vi "Read Config.vi"(8 "error in (no error)":errorcluster, 9 "Re-Init?":bool, 10 "ICM File In":path, 11 "Scaling in":refnum<class "Scaling.lvclass">) -> (0 "error out":errorcluster, 3 "Scaling out":refnum<class "Scaling.lvclass">)   [LabVIEW 2018, in "Scaling.lvclass"]
doc: "Scaling.lvclass:Read Config.vi\n\nThis is the template for the Read Config VI for the Scaling class.\n\nInstrument Communication Module Version 1.0\nSeptember, 2017 Original Code Consulting David Thomson\n www.originalcode.com"
uses:
  Scaling.lvclass
  Scaling.lvclass/Scaling.ctl
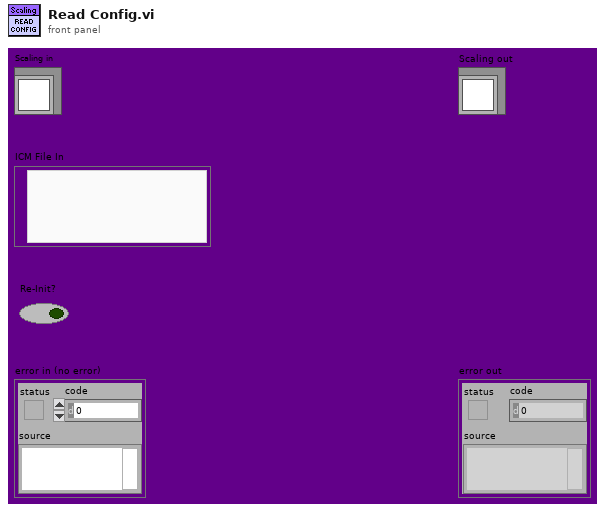
[diagram p1: front panel]
types:
  T1 = typedef "Scaling Def.ctl" = cluster{"Channel":string, "Scaling":string, "Instance":string}
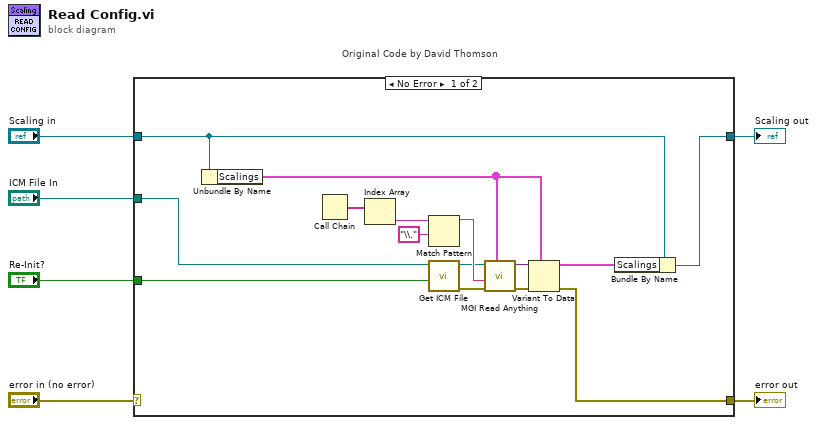
[diagram p0: block diagram]
diagram:
  n1 = case "Original Code by David Thomson" shown="No Error" "error in (no error)" {
    selector: "error in (no error)" -> [_ w23]
    tunnel: [w7 w23] -> w5
    tunnel: [w8 w22] -> w3
    tunnel: "Scaling in" -> [w9 w22]
    tunnel: "ICM File In" -> [w12 _]
    tunnel: "Re-Init?" -> [w11 _]
    frame No Error {
      n2 = Unbundle By Name(w9) -> ("Scalings"=w13:T1[])
      n3 = Call Chain() -> (call chain=w17:string[])
      n4 = Index Array(array=w17) -> (element=w16:string)  [unwired: 1 in]
      n5 = Match Pattern(string=w16, regular expression="\\.") -> (before substring=w19:string)  [unwired: 1 in, 3 out]
      n6 = call "Get ICM File.vi"("Re-Init?"=w11, "ICM File In"=w12) -> ("error out"=w15:errorcluster, "ICM File"=w14:path)  [unwired: 8 in]
      n7 = call <userlib>:"MGI Read Anything.vi"("Type of Anything"=w13, "Error In"=w15, "Section Name (Name of \"Type of Anything\")"=w19, "Path (dialog)"=w14) -> ("Error Out"=w21:errorcluster, "Anything"=w20:variant)  [unwired: 4 in, 2 out]
      n8 = Variant To Data(error in=w21, type=w13, Variant=w20) -> (data=w10:T1[], error out=w7:errorcluster)
      n9 = Bundle By Name(cluster=w9, "Scalings"=w10) -> (w8:refnum<class "Scaling.lvclass">)
    }
    frame Error {
    }
  }
  "error out" <- w5
  "Scaling out" <- w3
